vi "DataStream_U32.vi"(3 "error in (no error)":errorcluster, 4 "BytesToCombine":i32=4, 5 "data buffer":u8[](array[numeric]) format="%02x") -> (0 "error out":errorcluster, 1 "Debug Data":cluster{"4byte word":u8[], "word":u32}[](array[cluster]), 2 "32bit data":u32[](array[numeric]) format="%08x")   [LabVIEW 2010, in "lib1299.lvlib"]
uses:
  lib1299.lvlib
panel:
  in  "Debug data constant":cluster{"4byte word":u8[], "word":u32}
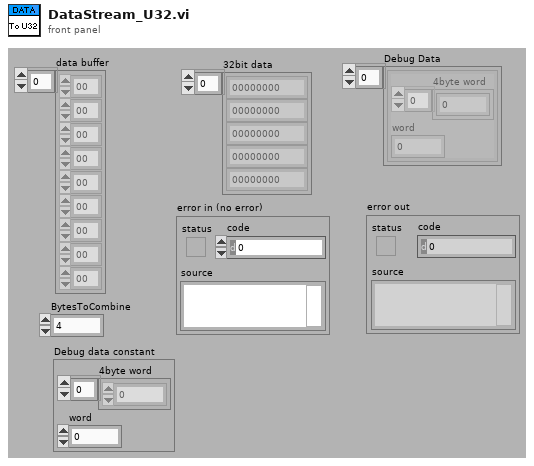
[diagram p1: front panel]
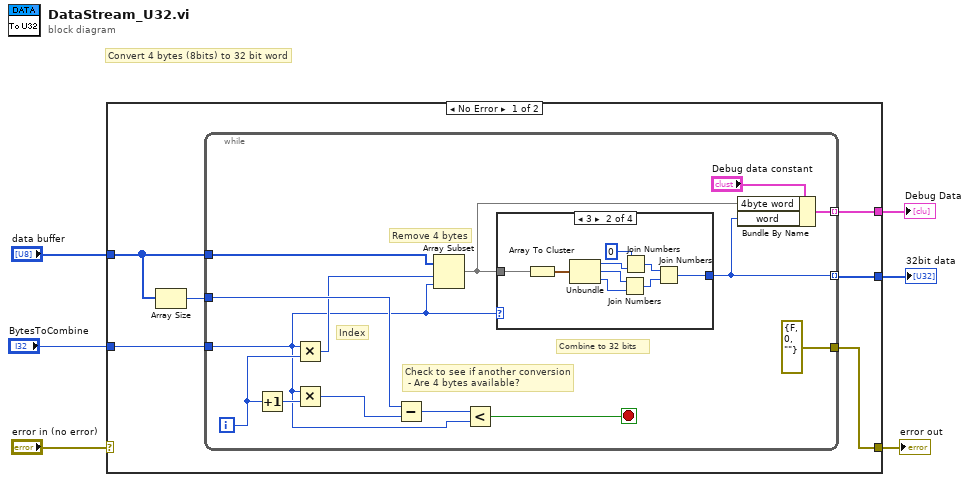
[diagram p0: block diagram]
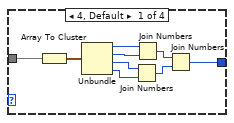
[diagram p2: hidden frame]
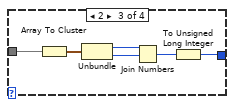
[diagram p3: hidden frame]
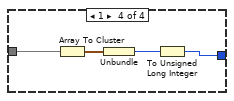
[diagram p4: hidden frame]
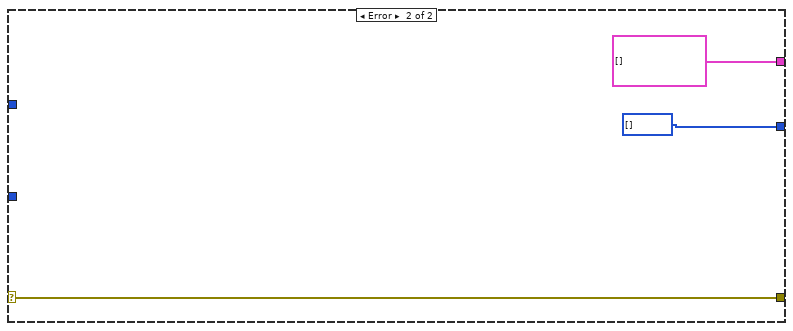
[diagram p5: hidden frame]
diagram:
  # "Convert 4 bytes (8bits) to 32 bit word"
  n1 = case shown="No Error" "error in (no error)" {
    selector: "error in (no error)" -> [_ w57]
    tunnel: "data buffer" -> [w12 _]
    tunnel: [w9 u32[] []] -> w5
    tunnel: [w10 w57] -> w3
    tunnel: [w8 cluster{"4byte word":u8[], "word":u32}[] []] -> w2
    tunnel: "BytesToCombine" -> [w7 _]
    frame No Error {
      n2 = Array Size(array=w12) -> (size(s)=w11:i32)
      n3 = while {
        tunnel: [w15] -> w9 mode=indexing
        tunnel: w12 -> [w25]
        tunnel: w11 -> [w24]
        tunnel: [errorcluster {"status"=FALSE, "code"=0, "source"=""} ("error IO")] -> w10
        tunnel: [w14] -> w8 mode=indexing
        tunnel: w7 -> [w13]
        i -> [w18]
        stop <- w26 stop-if-true
        # "Combine to 32 bits"
        # "Check to see if another conversion\n - Are 4 bytes available?"
        # "Remove 4 bytes"
        # "Index"
        n4 = Increment(x=w18) -> (x+1=w19:i32)
        n5 = Multiply(x=w13, y=w18) -> (x*y=w22:i32)
        n6 = Multiply(x=w13, y=w19) -> (x*y=w20:i32)
        n7 = Subtract(x=w24, y=w20) -> (x-y=w23:i32)
        n8 = Array Subset(array=w25, index=w22, length=w13) -> (w16:u8[])
        n9 = Less?(x=w23, y=w13) -> (x < y?=w26:bool)
        n10 = case shown="3" w13 {
          tunnel: w16 -> [w28 w41 w49 w54]
          tunnel: [w27 w40 w46 w51] -> w15
          frame 4, Default {
            n11 = Array To Cluster(array=w28) -> (cluster=w35:cluster{"[0]":u8, "[1]":u8, "[2]":u8, "[3]":u8})
            n12 = Unbundle(w35) -> ("[0]"=w29:u8, "[1]"=w34:u8, "[2]"=w33:u8, "[3]"=w32:u8)
            n13 = Join Numbers(hi=w33, lo=w32) -> ((hi.lo)=w30:u16)
            n14 = Join Numbers(hi=w29, lo=w34) -> ((hi.lo)=w31:u16)
            n15 = Join Numbers(hi=w31, lo=w30) -> ((hi.lo)=w27:u32)
          }
          frame 3 {
            n16 = Array To Cluster(array=w41) -> (cluster=w44:cluster{"[0]":u8, "[1]":u8, "[2]":u8})
            n17 = Unbundle(w44) -> ("[0]"=w37:u8, "[1]"=w38:u8, "[2]"=w39:u8)
            n18 = Join Numbers(hi=w38, lo=w39) -> ((hi.lo)=w42:u16)
            n19 = Join Numbers(hi=u8 0, lo=w37) -> ((hi.lo)=w43:u16)
            n20 = Join Numbers(hi=w43, lo=w42) -> ((hi.lo)=w40:u32)
          }
          frame 2 {
            n21 = Array To Cluster(array=w49) -> (cluster=w50:cluster{"[0]":u8, "[1]":u8})
            n22 = Unbundle(w50) -> ("[0]"=w48:u8, "[1]"=w47:u8)
            n23 = Join Numbers(hi=w48, lo=w47) -> ((hi.lo)=w45:u16)
            n24 = To Unsigned Long Integer(number=w45) -> (unsigned 32bit integer=w46:u32)
          }
          frame 1 {
            n25 = Array To Cluster(array=w54) -> (cluster=w53:cluster{"[0]":u8})
            n26 = Unbundle(w53) -> ("[0]"=w52:u8)
            n27 = To Unsigned Long Integer(number=w52) -> (unsigned 32bit integer=w51:u32)
          }
        }
        n28 = Bundle By Name(cluster="Debug data constant", "4byte word"=w16, "word"=w15) -> (w14:cluster{"4byte word":u8[], "word":u32})
      }
    }
    frame Error {
    }
  }
  "32bit data" <- w5
  "error out" <- w3
  "Debug Data" <- w2
